vi "Oscilloscope.vi"() -> ()   [LabVIEW 2016]
uses:
  controls/Enum.ctl
  <vilib>/measure/masml.llb/ma_sml_Averaging Parameters.ctl
  <vilib>/measure/masml.llb/ma_sml_Averaging Settings.ctl
  <vilib>/addons/Spectral Measurements Toolset/LVSupport/SMT BZ spectrum settings.ctl
  <vilib>/rvi/errors/niLvFpgaAdjustHostInterfaceError.vi
  <vilib>/addons/Spectral Measurements Toolset/LVSupport/SMT Zoom Power Spectrum (WDT).vi
  <vilib>/rvi/interface/common/niFpgaWaitOnOcc.vi
  <vilib>/measure/maspectr.llb/FFT Power Spectrum and PSD for 1 Chan.vi
  <vilib>/rvi/interface/nirviMethod/nirviMethod.xnode
  controls/FPGAVIreferenceTypeDef.ctl
  FPGA Bitfiles/qnmController797_usbRIO_controllerFPGAmu.lvbitx
  <vilib>/rvi/interface/nirviReadWriteControl/nirviReadWriteControl.xnode
  Course Project/support/Message Queue/Message Queue.lvlib
  <vilib>/rvi/errors/niLvFpgaMergeErrorWithErrorCode.vi
  <vilib>/measure/NI_MAPro.lvlib
  Course Project/support/User Event - Stop/User Event - Stop.lvlib
  <vilib>/addons/Spectral Measurements Toolset/niSMT.lvlib
  NiFpgaLv.dll
  <vilib>/FPGAPlugInAG/USB-7856R OEM/niLvFpga_ReadFifo_USB-7856R OEM.vi
  <vilib>/FPGAPlugInAG/USB-7856R OEM/niLvFpga_AcknowledgeIrq_USB-7856R OEM.vi
  <vilib>/FPGAPlugInAG/USB-7856R OEM/niLvFpga_ConfigureFifo_USB-7856R OEM.vi
  <vilib>/FPGAPlugInAG/USB-7856R OEM/niLvFpga_StartFifo_USB-7856R OEM.vi
panel:
  in  "k":bool=TRUE
  out "f":dbl
  in  "Cursor":bool
  out "Signal":waveform(dbl)(graph)
  in  "Save":bool
  in  "Time":dbl=1e-06 format="%#.0ps"
  in  "Tab Control":enum32{"PSD"}(tab)
  in  "Averaging parameters":T1={"mode"=2, "weighting mode"=1, "Averages"=3000} {"Averages" min=1; "weighting mode" items=["Linear", "Exponential"]; "mode" items=["No averaging", "Vector averaging", "RMS averaging", "Peak hold"]}
  in  "restart":bool
  in  "psd?":u16(ring)=1 items=["Power Spectrum", "PS Density"]
  in  "Window":u16(ring)=1 items=["None ", "Hanning", "Hamming", "Blackman-Harris", "Exact Blackman", "Blackman", "Flat Top", "4 Term B-Harris ", "7 Term B-Harris", "Low Sidelobe"]
  in  "impedance":dbl=50.0 format="%.0pohm"
  in  "rms pk":u16(ring) items=["rms", "pk"]
  in  "Units":u16(ring)=1 items=["V", "V^2", "W", "dBm", "dBW", "dBV", "dBmV", "dBuV"]
  in  "Linear weighting mode":u16(ring) items=["one shot", "auto restart one shot", "moving average", "continuous"]
  in  "Resolution":dbl=1000.0 format="%#.0pHz"
  in  "Span":dbl=200000.0 format="%#_3pHz"
  in  "Center":dbl=200000.0 format="%.3pHz"
  in  "Sampling Frequency":dbl=1000000.0 caption="Sampling" format="%_3pS"
  out "Zoom PSD":cluster{"f0":dbl, "df":dbl, "spectrum":dbl[]}(graph)
  in  "Points":u16=5000 format="%#_6f"
  in  "Type":u16(ring) items=["Signal", "PSD", "PSD zoom"]
  in  "Acquire":bool=TRUE caption="Enable"
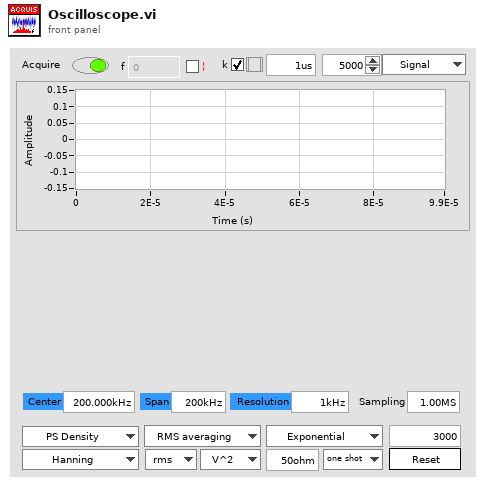
[diagram p1: front panel]
types:
  T1 = cluster{"mode":u16, "weighting mode":u16, "Averages":u32}
  T2 = typedef "Enum.ctl" = enum16{"Init", "Read", "Write"}
  T3 = typedef "Message Queue.lvlib/All Message Queues.ctl" = cluster{"IU":refnum<queue>}
  T4 = typedef "FPGAVIreferenceTypeDef.ctl" = refnum<k20>
  T5 = cluster{"hdt.int.s.transferSource":u8, "hdt.int.p.useInternalMemStartPos":bool, "hdt.int.p.memStartPos":fxp<+,14,14>, "hdt.int.p.readLength":u16, "hdt.int.p.readFwd":bool, "hdt.int.p.memReadDec":u16, "hdt.int.p.startTransfer":bool}
  T6 = enum16{"open", "replace", "create", "open or create", "replace or create", "replace or create with confirmation"}
  T7 = typedef "niSMT.lvlib/SMT BZ spectrum settings.ctl" = cluster{"center frequency":dbl, "span":dbl, "resolution bandwidth":dbl}
  T8 = cluster{"window":enum16{"None ", "Hanning", "Hamming", "Blackman-Harris", "Exact Blackman", "Blackman", "Flat Top", "4 Term B-Harris ", "7 Term B-Harris", "Low Sidelobe"}, "spectral lines":i32, "effective band specification":cluster{"fl":dbl, "fh":dbl}, "RBW definition":enum16{"3dB", "6dB", "ENBW", "bin width"}}
  T9 = typedef "NI_MAPro.lvlib/ma_sml_Averaging Parameters.ctl" = cluster{"averaging type":enum16{"no averaging", "vector averaging", "RMS averaging", "peak hold"}, "averaging settings":T10}
  T10 = typedef "NI_MAPro.lvlib/ma_sml_Averaging Settings.ctl" = cluster{"weighting type":enum16{"linear", "exponential"}, "weighting settings":cluster{"size":dbl, "linear weighting mode":enum16{"one shot", "auto restart one shot", "moving average", "continuous"}}}
  T11 = cluster{"units":enum16{"V", "V^2", "W", "dBm", "dBW", "dBV", "dBmV", "dBuV"}, "rms pk":enum16{"rms", "pk"}, "psd?":bool, "impedance(ohm)":dbl}
  T12 = typedef "niSMT.lvlib/SMT zoom settings.ctl" = cluster{"zoom FFT settings":T13, "frequency shift":dbl, "data format":enum16{"real", "complex modulated (array)", "complex modulated (interleaved)"}}
  T13 = typedef "NI_MAPro.lvlib/ma_sml_ND Zoom FFT Settings.ctl" = cluster{"zoom settings":cluster{"center frequency":dbl, "zoom":i32, "trim":dbl}, "FFT settings":cluster{"window":u16, "FFT size":i32}}
  T14 = typedef "NI_MAPro.lvlib/ma_sml_Spectral Info.ctl" = cluster{"spectrum type":enum16{"FFT Spectrum [complex]", "Amplitude [Magnitude]", "Power [Magnitude^2]", "Cross Spectrum [complex]", "Frequency Response [Complex]"}, "linear/dB":enum16{"linear", "dB"}, "window":u16, "window size":i32, "FFT size":i32}
  T15 = typedef "NI_MAPro.lvlib/ma_sml_Spectrum Cluster (real).ctl" = cluster{"f0":dbl, "df":dbl, "spectrum":dbl[]}
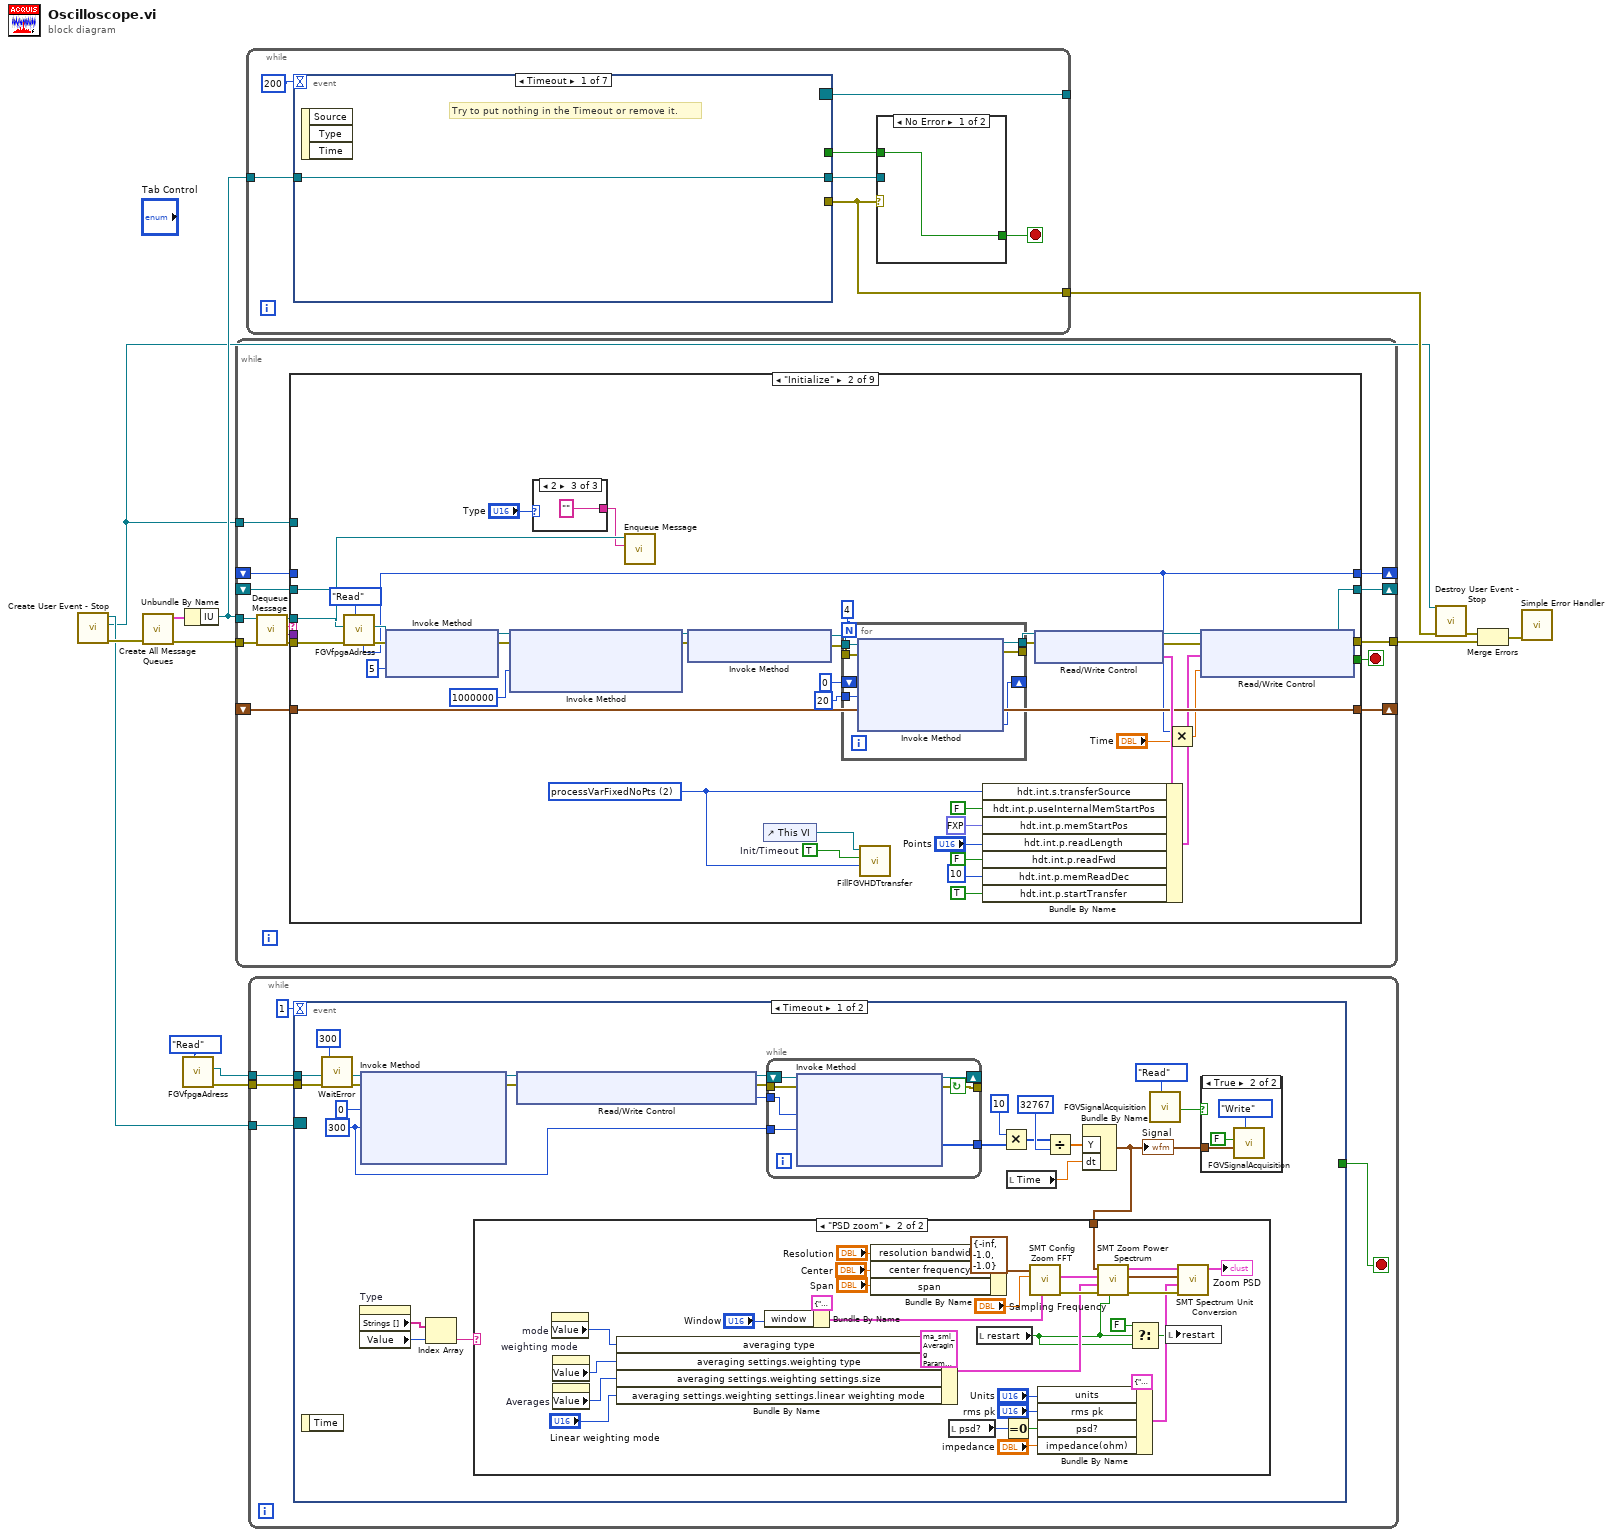
[diagram p0: block diagram]
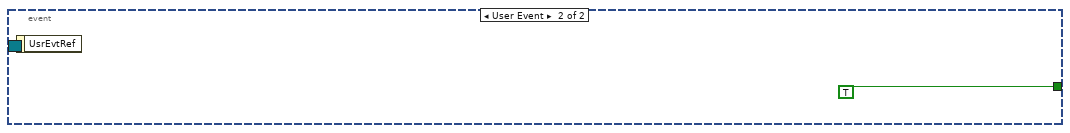
[diagram p4: hidden frame]
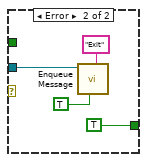
[diagram p5: hidden frame]
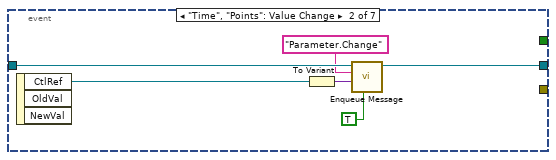
[diagram p6: hidden frame]
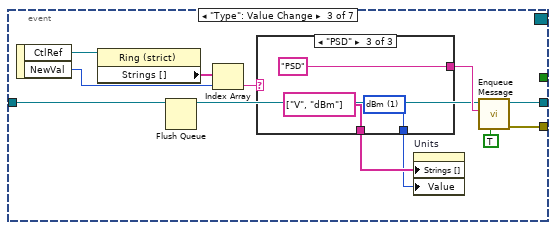
[diagram p7: hidden frame]
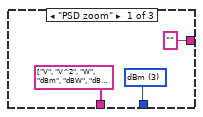
[diagram p8: hidden frame]
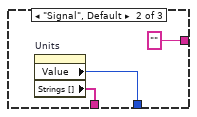
[diagram p9: hidden frame]
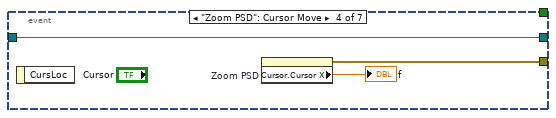
[diagram p10: hidden frame]
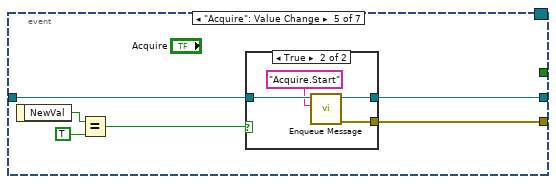
[diagram p11: hidden frame]
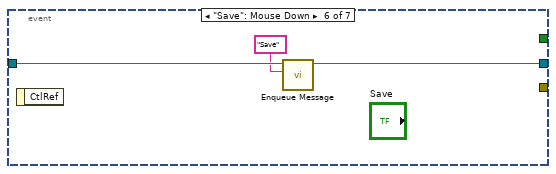
[diagram p13: hidden frame]
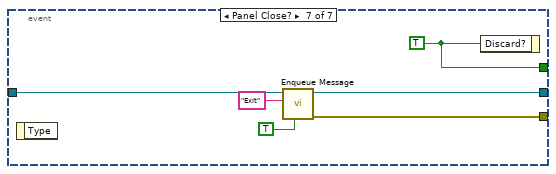
[diagram p14: hidden frame]
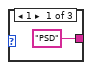
[diagram p16: hidden frame]
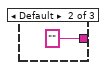
[diagram p17: hidden frame]
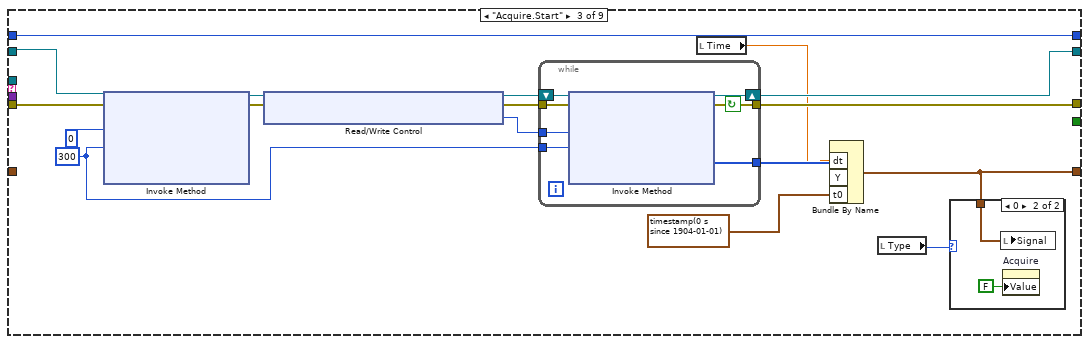
[diagram p18: hidden frame]
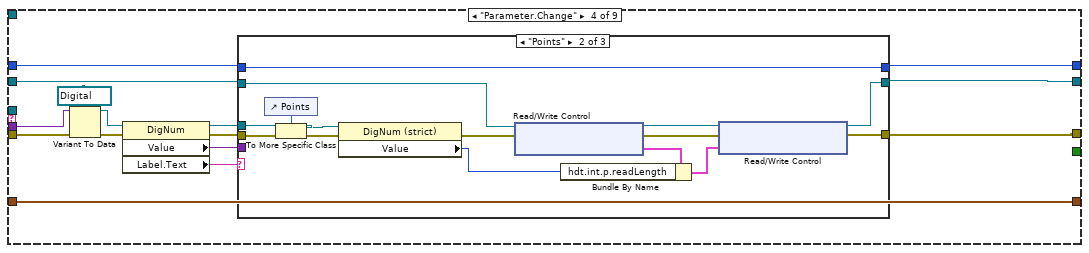
[diagram p20: hidden frame]
diagram:
  n1 = call "Create User Event - Stop.vi"() -> ("sortie d'erreur"=w5:errorcluster, "Événement utilisateur - Arrêt"=w1:refnum<user-event>, "Refnum Enregistrement à l'événement Arrêt"=w4:refnum<event-registration>)  [unwired: 9 in]
  n2 = call "Create All Message Queues.vi"("ErrorIn"=w5) -> ("ErrorOut"=w11:errorcluster, "MessageQueueOut"=w13:T3)  [unwired: 9 in]
  n3 = call "FGVfpgaAdress.vi"("Enum"=Enum."Read") -> ("error out"=w7:errorcluster, "FPGA VI Reference Out"=w6:T4)  [unwired: 5 in, 4 out]
  n4 = Unbundle By Name(w13) -> ("IU"=w12:refnum<queue>)
  n5 = while {
    tunnel: w12 -> [w22]
    tunnel: w11 -> [w26]
    tunnel: [w27] -> w9
    shift-right: [w20] -> _
    shift-left: _ -> [w19]
    shift-right: [w18] -> _
    shift-left: _ -> [w17]
    shift-right: [w16] -> _
    shift-left: _ -> [w15]
    tunnel: w1 -> [w14]
    stop <- w28 stop-if-true
    n6 = call "Dequeue Message.vi"("entrée d'erreur (pas d'erreur)"=w26, "File d'attente de messages"=w22) -> ("sortie d'erreur"=w25:errorcluster, "Données de message"=w24:variant, "Message"=w21:string, "File d'attente de message dup."=w23:refnum<queue>)  [unwired: 6 in]
    n7 = case "Conditions des messages" shown="\"Initialize\"" w21 {
      selector: w21 -> [_ _ _ _ _ _ _ _ w339]
      tunnel: w23 -> [_ w42 _ _ _ w171 _ w332 _]
      tunnel: w25 -> [w32 w56 w98 w121 w157 w168 w260 w330 _]
      tunnel: [w32 w54 w85 w115 w157 w164 w259 w323 w337] -> w27
      tunnel: [_ _ _ _ _ _ _ TRUE _] -> w28
      tunnel: w24 -> [_ _ _ w122 _ _ _ _ _]
      tunnel: [w31 w55 w96 w117 w156 w170 w264 w329 w335] -> w20
      tunnel: w19 -> [w31 w36 w97 w118 w156 w170 w264 w329 w335]
      tunnel: [w30 w71 w87 w123 w155 w163 w263 w328 w334] -> w18
      tunnel: w17 -> [w30 w71 _ w123 w155 w163 w263 w328 w334]
      tunnel: [w29 w37 w84 w111 w154 w169 w262 w327 w333] -> w16
      tunnel: w15 -> [w29 _ w84 w112 w154 w169 w262 w327 w333]
      tunnel: w14 -> [_ _ _ _ _ _ _ w326 _]
      frame "--------- Initialization ---------" {
      }
      frame "Initialize" {
        w35 = TRUE  # Init/Timeout
        w33 = u8 2 items=["memoryChan1", "memoryChan2", "processVarFixedNoPts", "processVarStream"] ("hdt.int.s.transferSource")
        n8 = call "FGVfpgaAdress.vi"("Enum"=Enum."Read", "error in"=w56, "FPGA VI Reference In"=w36) -> ("error out"=w69:errorcluster, "FPGA VI Reference Out"=w70:T4, "ioFreqHzOut"=w37:u32)  [unwired: 3 in, 3 out]
        n9 = xnode "Invoke Method"("FPGA VI Reference In"=w70, "error in"=w69, "IRQ Number(s)"=5) -> ("FPGA VI Reference Out"=w67:T4, "error out"=w66:errorcluster)
        n10 = xnode "Invoke Method"("FPGA VI Reference In"=w67, "error in"=w66, "Requested Depth"=u32 1000000) -> ("FPGA VI Reference Out"=w62:T4, "error out"=w64:errorcluster)  [unwired: 1 out]
        n11 = case shown="2" "Type" {
          tunnel: ["PSD" ("Message") "" ("Message") "" ("Message")] -> w40
          frame 1 {
          }
          frame Default {
          }
          frame 2 {
          }
        }
        n12 = call "Enqueue Message.vi"("Message"=w40, "Queue"=w42) -> ()  [unwired: 8 in, 2 out]
        n13 = xnode "Invoke Method"("FPGA VI Reference In"=w62, "error in"=w64) -> ("FPGA VI Reference Out"=w61:T4, "error out"=w58:errorcluster)
        n14 = control-ref of="This VI"() -> (w34:refnum<vi>)
        n15 = for {
          N: 4 -> [_]
          shift-right: [w77] -> _
          shift-left: u32 0 ("Elements Remaining") -> [w78]
          tunnel: 20 ("Timeout (ms)") -> [w76]
          tunnel: w61 -> [w82]
          tunnel: [w80] -> w53
          tunnel: w58 -> [w81]
          tunnel: [w79] -> w52
          n16 = xnode "Invoke Method"("FPGA VI Reference In"=w82, "error in"=w81, "Number of Elements"=w78, "Timeout (ms)"=w76) -> ("FPGA VI Reference Out"=w80:T4, "error out"=w79:errorcluster, "Elements Remaining"=w77:u32)  [unwired: 1 out]
        }
        n17 = call "FillFGVHDTtransfer.vi"("hdt.int.s.transferSource"=w33, "Used"=w35, "VI in"=w34) -> ()  [unwired: 9 in]
        n18 = xnode ("Read/Write Control")("FPGA VI Reference In"=w53, "error in"=w52) -> ("FPGA VI Reference Out"=w50:T4, "error out"=w51:errorcluster, "hdt.int.p.readParams"=w72:T5)
        n19 = Bundle By Name(cluster=w72, "hdt.int.s.transferSource"=w33, "hdt.int.p.useInternalMemStartPos"=FALSE, "hdt.int.p.memStartPos"=fxp<+,14,14> 0.0, "hdt.int.p.readLength"="Points", "hdt.int.p.readFwd"=FALSE, "hdt.int.p.memReadDec"=u16 10, "hdt.int.p.startTransfer"=TRUE) -> (w43:T5)
        n20 = Multiply(x=w37, y="Time") -> (x*y=w38:dbl)
        n21 = xnode ("Read/Write Control")("FPGA VI Reference In"=w50, "error in"=w51, "hdt.int.p.readParams"=w43, "aio.i.samplingDecimation"=w38) -> ("FPGA VI Reference Out"=w55:T4, "error out"=w54:errorcluster)
      }
      frame "Acquire.Start" {
        w92 = 300 ("Timeout (ms)")
        n22 = xnode "Invoke Method"("FPGA VI Reference In"=w97, "error in"=w98, "Number of Elements"=u32 0, "Timeout (ms)"=w92) -> ("FPGA VI Reference Out"=w89:T4, "error out"=w88:errorcluster)  [unwired: 2 out]
        n23 = xnode "Read/Write Control"("FPGA VI Reference In"=w89, "error in"=w88) -> ("FPGA VI Reference Out"=w95:T4, "error out"=w94:errorcluster, "hdt.int.p.readParams.hdt.int.p.readLength"=w93:u16)
        n24 = while {
          tunnel: w93 -> [w105]
          tunnel: [w104] -> w91
          tunnel: w92 -> [w103]
          shift-right: [w108] -> w96
          shift-left: w95 -> [w107]
          tunnel: w94 -> [w106]
          tunnel: [w102] -> w85
          stop <- w102 continue-if-true
          n25 = xnode "Invoke Method"("FPGA VI Reference In"=w107, "error in"=w106, "Number of Elements"=w105, "Timeout (ms)"=w103) -> ("FPGA VI Reference Out"=w108:T4, "error out"=w102:errorcluster, "Data"=w104:i16[])  [unwired: 1 out]
        }
        n26 = local read "Time"() -> (w83:dbl)
        n27 = Bundle By Name("dt"=w83, "Y"=w91, "t0"=timestamp(0 s since 1904-01-01)) -> (w87:waveform(i16))  [unwired: 1 in]
        n28 = local read "Type"() -> (w86:u16)
        n29 = case shown="0" w86 {
          tunnel: w87 -> [_ w100]
          frame Default {
          }
          frame 0 {
            n30 = local write "Signal"(w100) -> ()
            n31 = property on="Acquire" class="Bool (strict)"("Value"=FALSE ("Data Acquisition")) -> ()  [unwired: 2 in, 2 out]
          }
        }
      }
      frame "Parameter.Change" {
        n32 = Variant To Data(error in=w121, type=refnum<vi> refnum ("CtlRef"), Variant=w122) -> (data=w120:refnum<vi>, error out=w119:errorcluster)
        n33 = property class="DigNum"(reference=w120, error in=w119) -> (reference out=w109:refnum<vi>, error out=w116:errorcluster, "Value"=w114:variant, "Label.Text"=w113:string)
        n34 = case shown="\"Points\"" w113 {
          tunnel: w118 -> [w134 w150 w153]
          tunnel: [w133 w149 w153] -> w117
          tunnel: w116 -> [w126 w140 w152]
          tunnel: [w132 w148 w152] -> w115
          tunnel: w114 -> [_ _ _]
          tunnel: w112 -> [w131 w143 w151]
          tunnel: [w131 w143 w151] -> w111
          tunnel: w109 -> [w125 w141 _]
          frame "Time" {
            n35 = control-ref of="Time"() -> (w129:refnum<vi>)
            n36 = To More Specific Class(target class=w129, reference=w125, error in=w126) -> (specific class reference=w128:refnum<vi>, error out=w127:errorcluster)
            n37 = property class="DigNum (strict)"(reference=w128, error in=w127) -> (error out=w135:errorcluster, "Value"=w124:dbl)  [unwired: 1 out]
            n38 = Multiply(x=w131, y=w124) -> (x*y=w130:dbl)
            n39 = xnode ("Read/Write Control")("FPGA VI Reference In"=w134, "error in"=w135, "aio.i.samplingDecimation"=w130) -> ("FPGA VI Reference Out"=w133:T4, "error out"=w132:errorcluster)
          }
          frame "Points" {
            n40 = control-ref of="Points"() -> (w142:refnum<vi>)
            n41 = To More Specific Class(target class=w142, reference=w141, error in=w140) -> (specific class reference=w139:refnum<vi>, error out=w138:errorcluster)
            n42 = property class="DigNum (strict)"(reference=w139, error in=w138) -> (error out=w137:errorcluster, "Value"=w136:u16)  [unwired: 1 out]
            n43 = xnode ("Read/Write Control")("FPGA VI Reference In"=w150, "error in"=w137) -> ("FPGA VI Reference Out"=w146:T4, "error out"=w147:errorcluster, "hdt.int.p.readParams"=w145:T5)
            n44 = Bundle By Name(cluster=w145, "hdt.int.p.readLength"=w136) -> (w144:T5)
            n45 = xnode ("Read/Write Control")("FPGA VI Reference In"=w146, "error in"=w147, "hdt.int.p.readParams"=w144) -> ("FPGA VI Reference Out"=w149:T4, "error out"=w148:errorcluster)
          }
          frame Default {
          }
        }
      }
      frame "Type.Change" {
      }
      frame "PSD" {
        w161 = u16 1 items=["Signal", "PSD", "PSD zoom"] ("Type")
        n46 = local read "Type"() -> (w162:u16)
        n47 = Equal?(x=w162, y=w161) -> (x = y?=w160:bool)
        n48 = case shown="True" w160 {
          tunnel: w171 -> [_ w176]
          tunnel: w168 -> [w172 w175]
          tunnel: [w172 w174] -> w165
          frame False {
          }
          frame True {
            n49 = call "Enqueue Message.vi"("error in"=w175, "Message"="PSD", "Queue"=w176) -> ("error out"=w174:errorcluster)  [unwired: 7 in, 1 out]
          }
        }
        n50 = local read "Signal"() -> (w159:waveform(dbl))
        n51 = call "FGVSignalAcquisition.vi"("Enum"=Enum."Read", "error in"=w165) -> ("error out"=w166:errorcluster, "ReadOut"=w158:bool)  [unwired: 7 in, 1 out]
        n52 = case shown="True" w158 {
          tunnel: w166 -> [w177 w192]
          tunnel: [w177 w191] -> w164
          tunnel: w159 -> [_ w182]
          frame False {
          }
          frame True {
            n53 = local read "Units"() -> (w179:u16)
            n54 = local read "Window"() -> (w181:u16)
            n55 = Not Equal To 0?(x=w179) -> (x != 0?=w178:bool)
            n56 = call-poly <vilib>:"FFT Power Spectrum and PSD.vi"("export mode"="psd?", "averaging parameters"="Averaging parameters", "restart averaging (F)"="restart", "error in (no error)"=w192, "dB On (F)"=w178, "window"=w181, "time signal"=w182) -> ("error out"=w189:errorcluster, "Power Spectrum / PSD"=w180:cluster{"f0":dbl, "df":dbl, "magnitude":dbl[]})  [unwired: 1 in, 2 out]
            n57 = local write "Zoom PSD"(w180) -> ()
            n58 = Select(t=FALSE, s="restart", f="restart") -> (s? t:f=w185:bool)
            n59 = local write "restart"(w185) -> ()
            n60 = call "FGVSignalAcquisition.vi"("Enum"=Enum."Write", "error in"=w189, "DataIn"=w182, "ReadIn"=TRUE) -> ("error out"=w191:errorcluster)  [unwired: 5 in, 2 out]
          }
        }
      }
      frame "Save" {
        (unwired) 6 ("dimension size")
        w196 = T6."open or create" ("operation (0:open)")
        n61 = property on="rms pk" class="Ring (strict)"() -> ("Label.Text"=w237:string, "Strings []"=w231:string[], "Value"=w209:u16)  [unwired: 2 in, 2 out]
        n62 = property on="Units" class="Ring (strict)"() -> ("Label.Text"=w236:string, "Strings []"=w208:string[], "Value"=w207:u16)  [unwired: 2 in, 2 out]
        n63 = property on="Time" class="DigNum (strict)"() -> ("Label.Text"=w247:string, "Value"=w254:dbl)  [unwired: 2 in, 2 out]
        n64 = property on="Points" class="DigNum (strict)"() -> ("Label.Text"=w246:string, "Value"=w253:u16)  [unwired: 2 in, 2 out]
        n65 = property on="Center" class="DigNum (strict)"() -> ("Label.Text"=w245:string, "Value"=w252:dbl)  [unwired: 2 in, 2 out]
        n66 = property on="Resolution" class="DigNum (strict)"() -> ("Label.Text"=w244:string, "Value"=w251:dbl)  [unwired: 2 in, 2 out]
        n67 = property on="Span" class="DigNum (strict)"() -> ("Label.Text"=w243:string, "Value"=w250:dbl)  [unwired: 2 in, 2 out]
        n68 = property on="Sampling Frequency" class="DigNum (strict)"() -> ("Label.Text"=w242:string, "Value"=w249:dbl)  [unwired: 2 in, 2 out]
        n69 = property on="impedance" class="DigNum (strict)"() -> ("Label.Text"=w241:string, "Value"=w248:dbl)  [unwired: 2 in, 2 out]
        n70 = Index Array(array=w231, index=w209) -> (element=w210:string)
        n71 = Index Array(array=w208, index=w207) -> (element=w206:string)
        n72 = property on="mode" class="Ring (strict)"() -> ("Label.Text"=w238:string, "Strings []"=w232:string[], "Value"=w198:u16)  [unwired: 2 in, 2 out]
        n73 = Build Array(w247, w246, w245, w244, w243, w242, w241) -> (w230:string[])
        n74 = Build Array(w254, w253, w252, w251, w250, w249, w248) -> (w229:dbl[])
        n75 = property on="psd?" class="Ring (strict)"() -> ("Label.Text"=w239:string, "Strings []"=w233:string[], "Value"=w199:u16)  [unwired: 2 in, 2 out]
        n76 = property on="Linear weighting mode" class="Ring (strict)"() -> ("Label.Text"=w240:string, "Strings []"=w234:string[], "Value"=w201:u16)  [unwired: 2 in, 2 out]
        n77 = property on="weighting mode" class="Ring (strict)"() -> ("Label.Text"=w235:string, "Strings []"=w205:string[], "Value"=w204:u16)  [unwired: 2 in, 2 out]
        n78 = Index Array(array=w232, index=w198) -> (element=w197:string)
        n79 = Index Array(array=w233, index=w199) -> (element=w200:string)
        n80 = Index Array(array=w234, index=w201) -> (element=w202:string)
        n81 = Index Array(array=w205, index=w204) -> (element=w203:string)
        n82 = for {
          tunnel: w230 -> [w318] mode=indexing
          tunnel: w229 -> [w317] mode=indexing
          shift-right: [w315] -> w211
          shift-left: "" -> [w316]
          n83 = Number To Decimal String(number=w317) -> (decimal integer string=w320:string)  [unwired: 1 in]
          n84 = Concatenate Strings(w316, w318, "\t", w320, "\n") -> (w315:string)
        }
        n85 = Build Array(w240, w239, w238, w237, w236, w235) -> (w195:string[])
        n86 = Build Array(w202, w200, w197, w210, w206, w203) -> (w194:string[])
        n87 = disable-structure shown="Enabled" {
          disable-tunnel: [w296 _] -> w225
          frame Enabled {
            n88 = local read "Zoom PSD"() -> (w300:cluster{"f0":dbl, "df":dbl, "spectrum":dbl[]})
            n89 = property on="Center" class="DigNum (strict)"() -> ("Value"=w293:dbl)  [unwired: 2 in, 2 out]
            n90 = property on="Span" class="DigNum (strict)"() -> ("Value"=w295:dbl)  [unwired: 2 in, 2 out]
            n91 = Unbundle By Name(w300) -> ("spectrum"=w288:dbl[])
            n92 = Divide(x=w295, y=2.0) -> (x/y=w292:dbl)
            n93 = property on="Span" class="DigNum (strict)"() -> ("Value"=w290:dbl)  [unwired: 2 in, 2 out]
            n94 = Subtract(x=w293, y=w292) -> (x-y=w291:dbl)
            n95 = Array Size(array=w288) -> (size(s)=w287:i32)
            n96 = Divide(x=w290, y=w287) -> (x/y=w286:dbl)
            n97 = for {
              N: w287 -> [_]
              tunnel: w291 -> [w303]
              tunnel: w286 -> [w304]
              tunnel: [w301] -> w289 mode=indexing
              i -> [w305]
              n98 = Multiply(x=w304, y=w305) -> (x*y=w302:dbl)
              n99 = Add(x=w302, y=w303) -> (x+y=w301:dbl)
            }
            n100 = Build Array(w289, w288) -> (w299:dbl[][])
            n101 = Transpose 2D Array(2D array=w299) -> (transposed array=w298:dbl[][])
            n102 = Array To Spreadsheet String(array=w298, 3:"%.9e" ("format string")) -> (spreadsheet string=w296:string)  [unwired: 1 in]
          }
          frame Disabled {
          }
        }
        n103 = for {
          tunnel: w195 -> [w312] mode=indexing
          tunnel: w194 -> [w311] mode=indexing
          shift-right: [w310] -> w193
          shift-left: _ -> [w309]
          n104 = Concatenate Strings(w309, w312, "\t", w311, "\n") -> (w310:string)
        }
        n105 = property on="Points" class="DigNum (strict)"() -> ("Value"=w221:u16)  [unwired: 2 in, 2 out]
        n106 = property on="Time" class="DigNum (strict)"() -> ("Value"=w222:dbl)  [unwired: 2 in, 2 out]
        n107 = local read "Signal"() -> (w261:waveform(dbl))
        n108 = for {
          N: w221 -> [_]
          tunnel: w222 -> [w307]
          tunnel: [w306] -> w220 mode=indexing
          i -> [w308]
          n109 = Multiply(x=w307, y=w308) -> (x*y=w306:dbl)
        }
        n110 = Unbundle By Name(w261) -> ("Y"=w223:dbl[])
        n111 = Concatenate Strings(w211, w193, "X" ("string"), "\t", "Y" ("string"), "\n") -> (w212:string)
        n112 = Build Array(w220, w223) -> (w227:dbl[][])
        n113 = Open/Create/Replace File(error in=w260, operation (0:open)=w196) -> (refnum out=w255:refnum<file>, error out=w256:errorcluster)  [unwired: 4 in, 1 out]
        n114 = Write to Text File(file (use dialog)=w255, text=w212, error in=w256) -> (refnum out=w265:refnum<file>, error out=w257:errorcluster)  [unwired: 1 in, 1 out]
        n115 = Transpose 2D Array(2D array=w227) -> (transposed array=w226:dbl[][])
        n116 = Array To Spreadsheet String(array=w226, 3:"%.9e" ("format string")) -> (spreadsheet string=w224:string)  [unwired: 1 in]
        n117 = Write to Text File(file (use dialog)=w265, text=w224, error in=w257) -> (refnum out=w219:refnum<file>, error out=w218:errorcluster)  [unwired: 1 in, 1 out]
        n118 = Close File(refnum=w219, error in=w218) -> (error out=w213:errorcluster)  [unwired: 1 out]
        n119 = disable-structure shown="Enabled" {
          disable-tunnel: [w276 w285] -> w259
          disable-tunnel: w225 -> [w275 _]
          disable-tunnel: w212 -> [w271 _]
          disable-tunnel: w213 -> [w270 w285]
          disable-tunnel: w196 -> [w266 _]
          frame Enabled {
            n120 = Open/Create/Replace File(error in=w270, operation (0:open)=w266) -> (refnum out=w272:refnum<file>, error out=w273:errorcluster)  [unwired: 4 in, 1 out]
            n121 = case shown="True" "k" {
              tunnel: [w282 w283] -> w277
              tunnel: [w281 w284] -> w274
              tunnel: w273 -> [w280 w283]
              tunnel: w272 -> [w279 w284]
              tunnel: w271 -> [w278 _]
              frame False {
                n122 = Write to Text File(file (use dialog)=w279, text=w278, error in=w280) -> (refnum out=w281:refnum<file>, error out=w282:errorcluster)  [unwired: 1 in, 1 out]
              }
              frame True {
              }
            }
            n123 = Write to Text File(file (use dialog)=w274, text=w275, error in=w277) -> (refnum out=w269:refnum<file>, error out=w268:errorcluster)  [unwired: 1 in, 1 out]
            n124 = Close File(refnum=w269, error in=w268) -> (error out=w276:errorcluster)  [unwired: 1 out]
          }
          frame Disabled {
          }
        }
      }
      frame "Exit" {
        n125 = call "Fire User Event - Stop.vi"("Événement utilisateur - Arrêt"=w326) -> ("sortie d'erreur"=w325:errorcluster)  [unwired: 10 in]
        n126 = Release Queue(queue=w332, error in (no error)=w330) -> (error out=w324:errorcluster)  [unwired: 1 in, 2 out]
        n127 = control-ref of="This VI"() -> (w322:refnum<vi>)
        n128 = call "EmptyFGVHDTtransfer.vi"("VI in"=w322) -> ()  [unwired: 11 in]
        n129 = Merge Errors(w325, w324) -> (w323:errorcluster)
      }
      frame Default {
        n130 = Format Into String(format string="The message\"%s\" received in the gestion loop is not valid" ("Texte de message d'erreur inconnu"), w339) -> (resulting string=w336:string)  [unwired: 2 in, 1 out]
        n131 = call <vilib>:"Error Cluster From Error Code.vi"("error message (\"\")"=w336, "error code (0)"=1 ("code d'erreur (0)")) -> ("error out"=w337:errorcluster)  [unwired: 7 in]
      }
    }
  }
  n132 = while {
    tunnel: w12 -> [w347]
    tunnel: [w343] -> w3
    tunnel: [w342] -> _
    stop <- w345 stop-if-true
    n133 = event shown="[0] Timeout" {
      selector: _ -> [_ _ _ _ _ _ _]
      dyn-events: [_ _ _ _ _ _ _] -> w342
      timeout: 200 -> [_ _ _ _ _ _ _]
      tunnel: [_ _ _ _ _ _ w403] -> w346
      tunnel: w347 -> [w353 w359 w362 w383 w389 w397 w402]
      tunnel: [_ _ w369 w382 w387 _ w401] -> w343
      tunnel: [w353 w358 w371 w383 w388 w396 w400] -> w344
      event Timeout {
        # "Try to put nothing in the Timeout or remove it."
        n134 = event-data() -> ()  [unwired: 1 in, 3 out]
      }
      event "Time", "Points": Value Change {
        n135 = event-data() -> ("CtlRef"=w355:refnum<vi>)  [unwired: 1 in, 2 out]
        n136 = To Variant(anything=w355) -> (Variant=w356:variant)
        n137 = call "Enqueue Message.vi"("Prioritary message"=TRUE, "Data"=w356, "Message"="Parameter.Change", "Queue"=w359) -> ("Queue dup."=w358:refnum<queue>)  [unwired: 6 in, 1 out]
      }
      event "Type": Value Change {
        n138 = event-data() -> ("CtlRef"=w367:refnum<vi>, "NewVal"=w365:u16)  [unwired: 1 in]
        n139 = property class="Ring (strict)"(reference=w367) -> ("Strings []"=w366:string[])  [unwired: 1 in, 2 out]
        n140 = Flush Queue(queue=w362) -> (queue out=w361:refnum<queue>)  [unwired: 1 in, 2 out]
        n141 = Index Array(array=w366, index=w365) -> (element=w364:string)
        n142 = case shown="\"PSD\"" w364 {
          tunnel: ["" ("Message") "" ("Message") "PSD" ("Message")] -> w370
          tunnel: [string[] ["V", "V^2", "W", "dBm", "dBW", "dBV", "dBmV", "dBuV"] ("Strings []") w376 string[] ["V", "dBm"] ("Strings []")] -> w363
          tunnel: [w372 w375 w378] -> w360
          frame "PSD zoom" {
            w372 = u16 3 items=["V", "V^2", "W", "dBm", "dBW", "dBV", "dBmV", "dBuV"] ("Units")
          }
          frame "Signal", Default {
            n143 = property on="Units" class="Ring (strict)"() -> ("Value"=w375:u16, "Strings []"=w376:string[])  [unwired: 2 in, 2 out]
          }
          frame "PSD" {
            w378 = u16 1 items=["V", "dBm"] ("Units")
          }
        }
        n144 = property on="Units" class="Ring (strict)"("Strings []"=w363, "Value"=w360) -> ()  [unwired: 2 in, 2 out]
        n145 = call "Enqueue Message.vi"("Prioritary message"=TRUE, "Message"=w370, "Queue"=w361) -> ("error out"=w369:errorcluster, "Queue dup."=w371:refnum<queue>)  [unwired: 7 in]
      }
      event "Zoom PSD": Cursor Move {
        n146 = event-data() -> ()  [unwired: 1 in, 1 out]
        n147 = property on="Zoom PSD" class="WFGraph (strict)"() -> (error out=w382:errorcluster, "Cursor.Cursor X"=→"f":dbl)  [unwired: 2 in, 1 out]
      }
      event "Acquire": Value Change {
        n148 = event-data() -> ("NewVal"=w385:bool)  [unwired: 1 in]
        n149 = Equal?(x=w385, y=TRUE) -> (x = y?=w384:bool)
        n150 = case shown="True" w384 {
          tunnel: w389 -> [w390 w394]
          tunnel: [w390 w392] -> w388
          tunnel: [_ w391] -> w387
          frame False {
          }
          frame True {
            n151 = call "Enqueue Message.vi"("Message"="Acquire.Start", "Queue"=w394) -> ("error out"=w391:errorcluster, "Queue dup."=w392:refnum<queue>)  [unwired: 8 in]
          }
        }
      }
      event "Save": Mouse Down {
        n152 = event-data() -> ()  [unwired: 1 in, 1 out]
        n153 = call "Enqueue Message.vi"("Message"="Save", "Queue"=w397) -> ("Queue dup."=w396:refnum<queue>)  [unwired: 8 in, 1 out]
      }
      event Panel Close? {
        w403 = TRUE ("Rejeter ?")
        n154 = event-data() -> ()  [unwired: 1 in, 1 out]
        n155 = call "Enqueue Message.vi"("Prioritary message"=TRUE ("Message prioritaire ? (F)"), "Message"="Exit", "Queue"=w402) -> ("error out"=w401:errorcluster, "Queue dup."=w400:refnum<queue>)  [unwired: 7 in]
        n156 = event-data ("Event Filter Node")("Discard?"=w403) -> ()  [unwired: 1 in, 1 out]
      }
    }
    n157 = case shown="No Error" w343 {
      tunnel: [w348 TRUE ("Rejeter ?")] -> w345
      tunnel: w346 -> [w348 _]
      tunnel: w344 -> [_ w351]
      frame No Error {
      }
      frame Error {
        n158 = call "Enqueue Message.vi"("Prioritary message"=TRUE ("Message prioritaire ? (F)"), "Message"="Exit", "Queue"=w351) -> ()  [unwired: 7 in, 2 out]
      }
    }
  }
  n159 = while {
    tunnel: w7 -> [w408]
    tunnel: w6 -> [w407]
    tunnel: w4 -> [w406]
    stop <- w405 stop-if-true
    n160 = event shown="[0] Timeout" {
      selector: w406 -> [_ _]
      dyn-events: _ -> [_ _]
      timeout: 1 -> [_ _]
      tunnel: w408 -> [w411 _]
      tunnel: w407 -> [w431 _]
      tunnel: [_ TRUE] -> w405
      event Timeout {
        w422 = 300 ("Timeout (ms)")
        n161 = event-data() -> ()  [unwired: 1 in, 1 out]
        n162 = call "WaitError.vi"("error in (no error)"=w411, "milliseconds to wait"=u32 300) -> ("error out"=w410:errorcluster)  [unwired: 9 in]
        n163 = property on="Type" class="Ring (strict)"() -> ("Strings []"=w429:string[], "Value"=w430:u16)  [unwired: 2 in, 2 out]
        n164 = xnode "Invoke Method"("FPGA VI Reference In"=w431, "error in"=w410, "Number of Elements"=u32 0, "Timeout (ms)"=w422) -> ("FPGA VI Reference Out"=w426:T4, "error out"=w425:errorcluster)  [unwired: 2 out]
        n165 = Index Array(array=w429, index=w430) -> (element=w428:string)
        n166 = xnode "Read/Write Control"("FPGA VI Reference In"=w426, "error in"=w425) -> ("FPGA VI Reference Out"=w423:T4, "error out"=w424:errorcluster, "hdt.int.p.readParams.hdt.int.p.readLength"=w421:u16)
        n167 = while {
          tunnel: [w438] -> w417
          tunnel: w422 -> [w437]
          shift-right: [w441] -> _
          shift-left: w423 -> [w440]
          tunnel: w424 -> [w439]
          tunnel: [w436] -> _
          tunnel: w421 -> [w435]
          stop <- w436 continue-if-true
          n168 = xnode "Invoke Method"("FPGA VI Reference In"=w440, "error in"=w439, "Number of Elements"=w435, "Timeout (ms)"=w437) -> ("FPGA VI Reference Out"=w441:T4, "error out"=w436:errorcluster, "Data"=w438:i16[])  [unwired: 1 out]
        }
        n169 = Multiply(x=10, y=w417) -> (x*y=w413:i32[])
        n170 = local read "Time"() -> (w418:dbl)
        n171 = Divide(x=w413, y=i16 32767) -> (x/y=w412:dbl[])
        n172 = Bundle By Name("Y"=w412, "dt"=w418) -> (w415:waveform(dbl))  [unwired: 1 in]
        "Signal" <- w415
        n173 = case shown="\"PSD zoom\"" w428 {
          tunnel: w415 -> [_ w468]
          frame "0", Default {
          }
          frame "PSD zoom" {
            n174 = property on="mode" class="Ring (strict)"() -> ("Value"=w458:u16)  [unwired: 2 in, 2 out]
            n175 = property on="weighting mode" class="Ring (strict)"() -> ("Value"=w459:u16)  [unwired: 2 in, 2 out]
            n176 = property on="Averages" class="DigNum (strict)"() -> ("Value"=w460:u32)  [unwired: 2 in, 2 out]
            n177 = Bundle By Name(cluster=T9 {"averaging type"=enum."no averaging", "averaging settings"={"weighting type"=enum."linear", "weighting settings"={"size"=10.0, "linear weighting mode"=enum."moving average"}}} ("averaging parameters 2"), "averaging type"=w458, "averaging settings.weighting type"=w459, "averaging settings.weighting settings.size"=w460, "averaging settings.weighting settings.linear weighting mode"="Linear weighting mode") -> (w453:T9)
            n178 = Bundle By Name(cluster=T8 {"window"=enum."7 Term B-Harris", "spectral lines"=-1, "effective band specification"={"fl"=0.0, "fh"=0.5}, "RBW definition"=enum."3dB"} ("advanced settings"), "window"="Window") -> (w456:T8)
            n179 = Bundle By Name(cluster=T7 {"center frequency"=-inf, "span"=-1.0, "resolution bandwidth"=-1.0} ("spectrum settings"), "resolution bandwidth"="Resolution", "center frequency"="Center", "span"="Span") -> (w450:T7)
            n180 = local read "psd?"() -> (w447:u16)
            n181 = local read "restart"() -> (w443:bool)
            n182 = Equal To 0?(x=w447) -> (x = 0?=w446:bool)
            n183 = call <vilib>:"SMT Config Zoom FFT.vi"("advanced settings"=w456, "fs"="Sampling Frequency", "spectrum settings"=w450) -> ("error out"=w473:errorcluster, "SMT zoom settings"=w448:T12)  [unwired: 5 in, 2 out]
            n184 = Bundle By Name(cluster=T11 {"units"=enum."dBV", "rms pk"=enum."pk", "psd?"=FALSE, "impedance(ohm)"=50.0} ("unit conversion settings"), "units"="Units", "rms pk"="rms pk", "psd?"=w446, "impedance(ohm)"="impedance") -> (w466:T11)
            n185 = call-poly <vilib>:"SMT Zoom Power Spectrum.vi"("restart averaging?"=w443, "error in (no error)"=w473, "averaging parameters"=w453, "SMT zoom settings"=w448, "signal in"=w468) -> ("error out"=w472:errorcluster, "spectral info"=w470:T14, "power spectrum"=w471:T15)  [unwired: 2 in, 2 out]
            n186 = Select(t=FALSE, s=w443, f=w443) -> (s? t:f=w445:bool)
            n187 = local write "restart"(w445) -> ()
            n188 = call <vilib>:"SMT Spectrum Unit Conversion.vi"("error in (no error)"=w472, "unit conversion settings"=w466, "spectral info in"=w470, "power spectrum"=w471) -> ("unit converted spectrum"=→"Zoom PSD":cluster{"f0":dbl, "df":dbl, "spectrum":dbl[]})  [unwired: 4 in, 3 out]
          }
        }
        n189 = call "FGVSignalAcquisition.vi"("Enum"=Enum."Read") -> ("ReadOut"=w419:bool)  [unwired: 8 in, 2 out]
        n190 = case shown="True" w419 {
          tunnel: w415 -> [_ w433]
          frame False {
          }
          frame True {
            n191 = call "FGVSignalAcquisition.vi"("Enum"=Enum."Write", "DataIn"=w433, "ReadIn"=FALSE) -> ()  [unwired: 6 in, 3 out]
          }
        }
      }
      event User Event {
        n192 = event-data() -> ()  [unwired: 1 in, 1 out]
      }
    }
  }
  n193 = call "Destroy User Event - Stop.vi"("entrée d'erreur (pas d'erreur)"=w3, "Événement utilisateur - Arrêt"=w1) -> ("sortie d'erreur"=w2:errorcluster)  [unwired: 9 in]
  n194 = Merge Errors(w2, w9) -> (w10:errorcluster)
  n195 = call <vilib>:"Simple Error Handler.vi"("error in (no error)"=w10) -> ()  [unwired: 4 in, 5 out]
